vi "Variant_BuildArrayFromElementArray.vi"(8 "error in (no error)":errorcluster, 9 "Dimensions":u32[](array[numeric]), 10 "Elements":variant[](array[variant]), 11 "Default Array":variant) -> (0 "error out":errorcluster, 3 "Output Array":variant)   [LabVIEW 2017, in "JSONtext.lvlib"]
uses:
  <vilib>/Utility/GetType.llb/Type Descriptor I16.ctl
  <vilib>/LabVIEW Open Source Project/Data Manipulation/TypeDescriptor/TypeDescriptor_GetType.vi
  <vilib>/LabVIEW Open Source Project/Data Manipulation/TypeDescriptor/TypeDescriptor_GetPString.vi
  <vilib>/Utility/GetType.llb/Get Type Code from I16 Array And Pos.vi
  <vilib>/Utility/GetType.llb/TD_Get Array Information.vi
  JSONtext.lvlib
  <vilib>/LabVIEW Open Source Project/Data Manipulation/Variant/OpenVariant.lvlib
  <vilib>/LabVIEW Open Source Project/Data Manipulation/TypeDescriptor/OpenDescriptor.lvlib
  <vilib>/Utility/VariantDataType/VariantType.lvlib
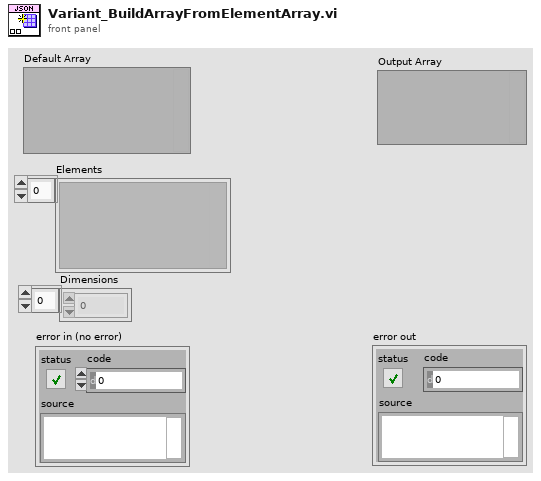
[diagram p1: front panel]
types:
  T1 = typedef "Type Descriptor I16.ctl" = i16
  T2 = typedef "VariantType.lvlib/Type.ctl" = enum8{"Invalid Type", "Void", "I8", "I16", "I32", "I64", "U8", "U16", "U32", "U64", "Single Float", "Double Float", "Extended Float", "Single Complex", "Double Complex", "Extended Complex", "Enum U8", "Enum U16", "Enum U32", "Enum U64", "Single Float With Unit", "Double Float With Unit", "Extended Float With Unit", "Single Complex with Unit", "Double Complex with Unit", "Extended Complex with Unit", "Boolean", "String", "Path", "Picture", "Tag", "Array", "Cluster", "Variant", "LV Variant", "Waveform", "Timestamp", "Digital Waveform", "Digital Data", "ExpressData", "Refnum", "External Data", "VI", "Poly VI", "LabVIEW Class Instance", "Fixed Point"}
  T3 = typedef "Type Descriptor I16 Array.ctl" = T1[]
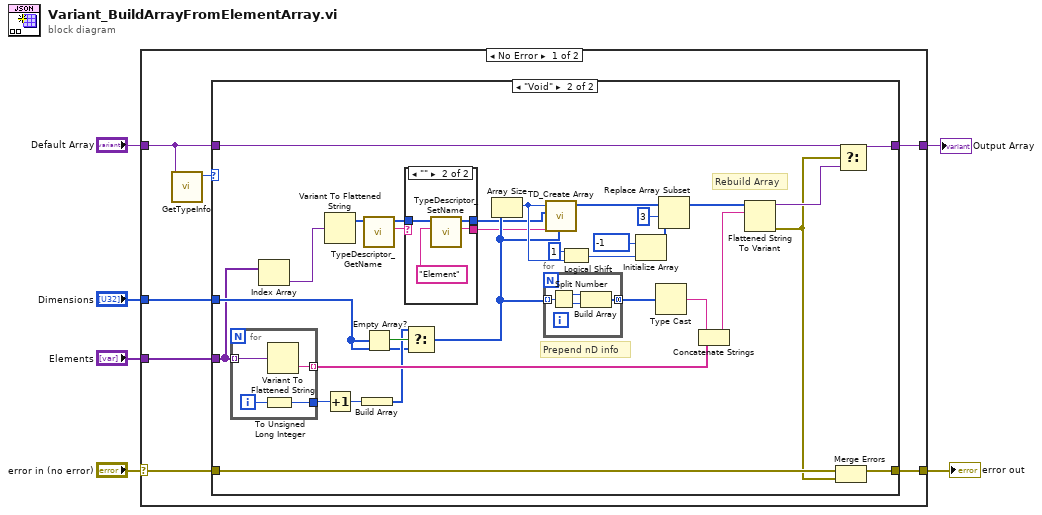
[diagram p0: block diagram]
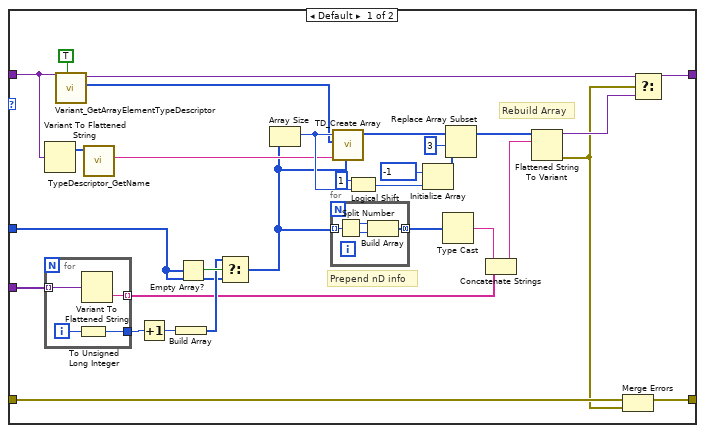
[diagram p2: hidden frame]
diagram:
  n1 = case shown="No Error" "error in (no error)" {
    selector: "error in (no error)" -> [w10 w98]
    tunnel: "Dimensions" -> [w13 _]
    tunnel: "Elements" -> [w9 _]
    tunnel: [w11 w98] -> w4
    tunnel: [w12 w97] -> w3
    tunnel: "Default Array" -> [w8 w97]
    frame No Error {
      n2 = call <vilib>:"GetTypeInfo.vi"("Variant"=w8) -> ("Type Enum"=w7:T2)  [unwired: 6 in, 4 out]
      n3 = case shown="\"Void\"" w7 {
        tunnel: w13 -> [w15 w60]
        tunnel: [w30 w70] -> w12
        tunnel: [w25 w68] -> w11
        tunnel: w10 -> [w24 w67]
        tunnel: w9 -> [w17 w58]
        tunnel: w8 -> [w22 w52]
        frame Default {
          # "Prepend nD info"
          # "Rebuild Array"
          n4 = Variant To Flattened String(Variant=w22) -> (1:w29:i16[])  [unwired: 1 out]
          n5 = for {
            tunnel: w17 -> [w47] mode=indexing
            tunnel: [w46] -> w16 mode=indexing
            tunnel: [w44] -> w21
            i -> [w45]
            n6 = To Unsigned Long Integer(number=w45) -> (unsigned 32bit integer=w44:u32)
            n7 = Variant To Flattened String(Variant=w47) -> (data string=w46:string)  [unwired: 1 out]
          }
          n8 = call <vilib>:"Variant_GetArrayElementTypeDescriptor.vi"("Name Element if empty string (F)"=TRUE, "Array"=w22) -> ("Element Descriptor"=w27:i16[], "Array dup"=w26:variant)  [unwired: 7 in, 1 out]
          n9 = call <vilib>:"TypeDescriptor_GetName.vi"("type descriptor"=w29) -> ("name"=w28:string)  [unwired: 8 in, 2 out]
          n10 = Increment(x=w21) -> (x+1=w20:u32)
          n11 = Build Array(w20) -> (w18:u32[])
          n12 = Empty Array?(array=w15) -> (empty?=w19:bool)
          n13 = Select(t=w18, s=w19, f=w15) -> (s? t:f=w14:u32[])
          n14 = Array Size(array=w14) -> (size(s)=w43:i32)
          n15 = for {
            tunnel: w14 -> [w51] mode=indexing
            tunnel: [w48] -> w38 mode=concatenating
            n16 = Split Number(x=w51) -> (hi(x)=w50:u16, lo(x)=w49:u16)
            n17 = Build Array(w50, w49) -> (w48:u16[])
          }
          n18 = call <vilib>:"TD_Create Array.vi"("Dim Lengths"=w14, "Name"=w28, "Array Elt"=w27, "N Dims"=w43) -> ("NewArray"=w34:T3)  [unwired: 7 in]
          n19 = Logical Shift(y=i16 1, x=w43) -> (x << y=w41:i32)
          n20 = Initialize Array(T1 -1 ("Numeric"), w41) -> (w37:T1[])
          n21 = Type Cast(x=w38) -> (*(type *) &x=w39:string)  [unwired: 1 in]
          n22 = Replace Array Subset(array=w34, new element=w37, index=3) -> (w35:T3)
          n23 = Concatenate Strings(w39, w16) -> (w42:string)
          n24 = Flattened String To Variant(6:w42, 7:w35) -> (0:w23:errorcluster, 3:w31:variant)  [unwired: 1 in]
          n25 = Merge Errors(w24, w23) -> (w25:errorcluster)
          n26 = Select(t=w26, s=w23, f=w31) -> (s? t:f=w30:variant)
        }
        frame "Void" {
          # "Prepend nD info"
          # "Rebuild Array"
          n27 = for {
            tunnel: w58 -> [w92] mode=indexing
            tunnel: [w91] -> w65 mode=indexing
            tunnel: [w89] -> w64
            i -> [w90]
            n28 = To Unsigned Long Integer(number=w90) -> (unsigned 32bit integer=w89:u32)
            n29 = Variant To Flattened String(Variant=w92) -> (data string=w91:string)  [unwired: 1 out]
          }
          n30 = Index Array(array=w58) -> (element=w57:variant)  [unwired: 1 in]
          n31 = Variant To Flattened String(Variant=w57) -> (1:w69:i16[])  [unwired: 1 out]
          n32 = Increment(x=w64) -> (x+1=w63:u32)
          n33 = Build Array(w63) -> (w61:u32[])
          n34 = call <vilib>:"TypeDescriptor_GetName.vi"("type descriptor"=w69) -> ("name"=w56:string, "type descriptor dup"=w54:i16[])  [unwired: 8 in, 1 out]
          n35 = Empty Array?(array=w60) -> (empty?=w62:bool)
          n36 = case shown="\"\"" w56 {
            selector: w56 -> [w84 _]
            tunnel: [w84 w87] -> w55
            tunnel: w54 -> [w83 w88]
            tunnel: [w83 w86] -> w53
            frame Default {
            }
            frame "" {
              n37 = call <vilib>:"TypeDescriptor_SetName.vi"("name"="Element", "type descriptor"=w88) -> ("name out"=w87:string, "type descriptor dup"=w86:i16[])  [unwired: 7 in, 1 out]
            }
          }
          n38 = Select(t=w61, s=w62, f=w60) -> (s? t:f=w59:u32[])
          n39 = Array Size(array=w59) -> (size(s)=w82:i32)
          n40 = for {
            tunnel: w59 -> [w96] mode=indexing
            tunnel: [w93] -> w77 mode=concatenating
            n41 = Split Number(x=w96) -> (hi(x)=w95:u16, lo(x)=w94:u16)
            n42 = Build Array(w95, w94) -> (w93:u16[])
          }
          n43 = call <vilib>:"TD_Create Array.vi"("Dim Lengths"=w59, "Name"=w55, "Array Elt"=w53, "N Dims"=w82) -> ("NewArray"=w73:T3)  [unwired: 7 in]
          n44 = Logical Shift(y=i16 1, x=w82) -> (x << y=w80:i32)
          n45 = Initialize Array(T1 -1 ("Numeric"), w80) -> (w76:T1[])
          n46 = Type Cast(x=w77) -> (*(type *) &x=w78:string)  [unwired: 1 in]
          n47 = Replace Array Subset(array=w73, new element=w76, index=3) -> (w74:T3)
          n48 = Concatenate Strings(w78, w65) -> (w81:string)
          n49 = Flattened String To Variant(6:w81, 7:w74) -> (0:w66:errorcluster, 3:w71:variant)  [unwired: 1 in]
          n50 = Merge Errors(w67, w66) -> (w68:errorcluster)
          n51 = Select(t=w52, s=w66, f=w71) -> (s? t:f=w70:variant)
        }
      }
    }
    frame Error {
    }
  }
  "error out" <- w4
  "Output Array" <- w3
